vi "InjA-RT.vi"() -> ()   [LabVIEW 2016]
uses:
  Common-Control/Aperture states.ctl
  Common-Control/GP307 cluster.ctl
  Common-Control/Glassman Control.ctl
  <vilib>/FPGAPlugInAG/cRIO-9074/niLvFpga_Open_cRIO-9074.vi
  <vilib>/Utility/error.llb/Error Cluster From Error Code.vi
  <vilib>/rvi/errors/niLvFpgaAdjustHostInterfaceError.vi
  <vilib>/rvi/interface/nirviOpenFPGA/nirviOpenFPGA.xnode
  FPGA Bitfiles/Controlsoftware2_FPGATarget7_InjA-FPGA_SFV0QsfDh2c.lvbitx
  InjA-FPGA.vi
  <vilib>/rvi/interface/nirviReadWriteControl/nirviReadWriteControl.xnode
  Common-Control/Aperture Readback.ctl
  <vilib>/Instr/_visa.llb/VISA Configure Serial Port (Instr).vi
  NiFpgaLv.dll
panel:
  in  "Tab Control":T1(tab)
  out "Y Steerer Monitor.V-monitor":fxp<+/-,16,5>
  out "Y Steerer Monitor.I-monitor":fxp<+/-,16,5>
  out "X Steerer Monitor.V-monitor":fxp<+/-,16,5>
  out "X Steerer Monitor.I-monitor":fxp<+/-,16,5>
  out "Einzel 1 Monitor.I-monitor":fxp<+/-,16,5>
  out "Einzel 1 Monitor.V-monitor":fxp<+/-,16,5>
  out "Einzel 2 Monitor.V-monitor":fxp<+/-,16,5>
  out "Einzel 2 Monitor.I-monitor":fxp<+/-,16,5>
  out "Y Steerer set":T2
  out "Einzel 2 set":T2
  out "X Steerer set":T2
  out "Einzel 1 set":T2
  out "InjA Vac Cluster":T3
  out "InjA Convectron":dbl
  out "InjA Ion Gauge":dbl
  out "Ion Gauge 1":u8[](array[numeric])
  out "Convectron 1":u8[](array[numeric])
  out "Ion Gauge 2":u8[](array[numeric])
  out "Convectron 2":u8[](array[numeric])
  out "Turbo Error Status":bool
  out "Turbo Rotation Status":bool
  out "Turbo Rotation Speed":dbl
  out "Vacuum Gauge interlock":bool
  out "Pre-Acc Image  Aperture Position 2":cluster{"IN sensor":bool, "OUT sensor":bool}
  out "Pre-Acc Image  Aperture Position":T4
  out "BPM 2":bool
  out "BPM 2 x10":bool
  out "Vac cluster loop error":errorcluster
  out "HV control loop error":errorcluster
  out "Turbo readback loop error":errorcluster
  out "HV readback loop error":errorcluster
  out "Acuator-Sensor loop error":errorcluster
  out "error out":errorcluster
  out "source cage Ion gauge Cluster 2":T5={"beam line pressure  Gauge "="9.90E+09\r\n", "Turbo convectorn Gauge "="0.00E+00\r\n", "Steerer Convectro Gauge "="2.40E-08\r\n", "Ion gauge2"="7.60E-01\r\n"}
  out "element":string="0.00E+00\r\n"
  out "read buffer":string="0.00E+00\r\n"
  out "Error Reporter":errorcluster
  in  "source cage Ion gauge Cluster 4":T5
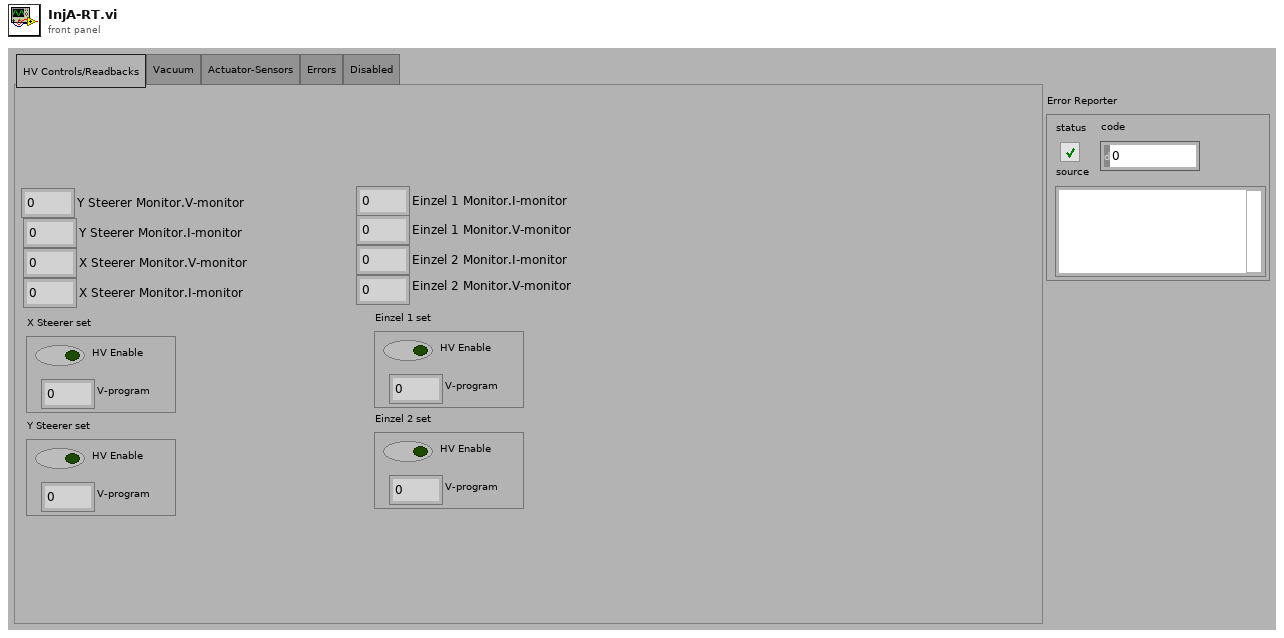
[diagram p1: front panel]
types:
  T1 = enum32{"HV Controls/Readbacks", "Vacuum", "Actuator-Sensors", "Errors", "Disabled"}
  T2 = typedef "Glassman Control.ctl" = cluster{"V-program":fxp<+/-,16,5>, "HV Enable":bool}
  T3 = typedef "GP307 cluster.ctl" = cluster{"Ion gauge 1":string, "Convectron  Gauge 1 ":string, "Ion Gauge 2":string, "Convectrom Gauge 2":string}
  T4 = typedef "Aperture states.ctl" = enum16{"Aperture status unclear", "Aperture in", "Aperture out"}
  T5 = cluster{"beam line pressure  Gauge ":string, "Turbo convectorn Gauge ":string, "Steerer Convectro Gauge ":string, "Ion gauge2":string}
  T6 = typedef "Aperture Readback.ctl" = cluster{"IN sensor":bool, "OUT sensor":bool}
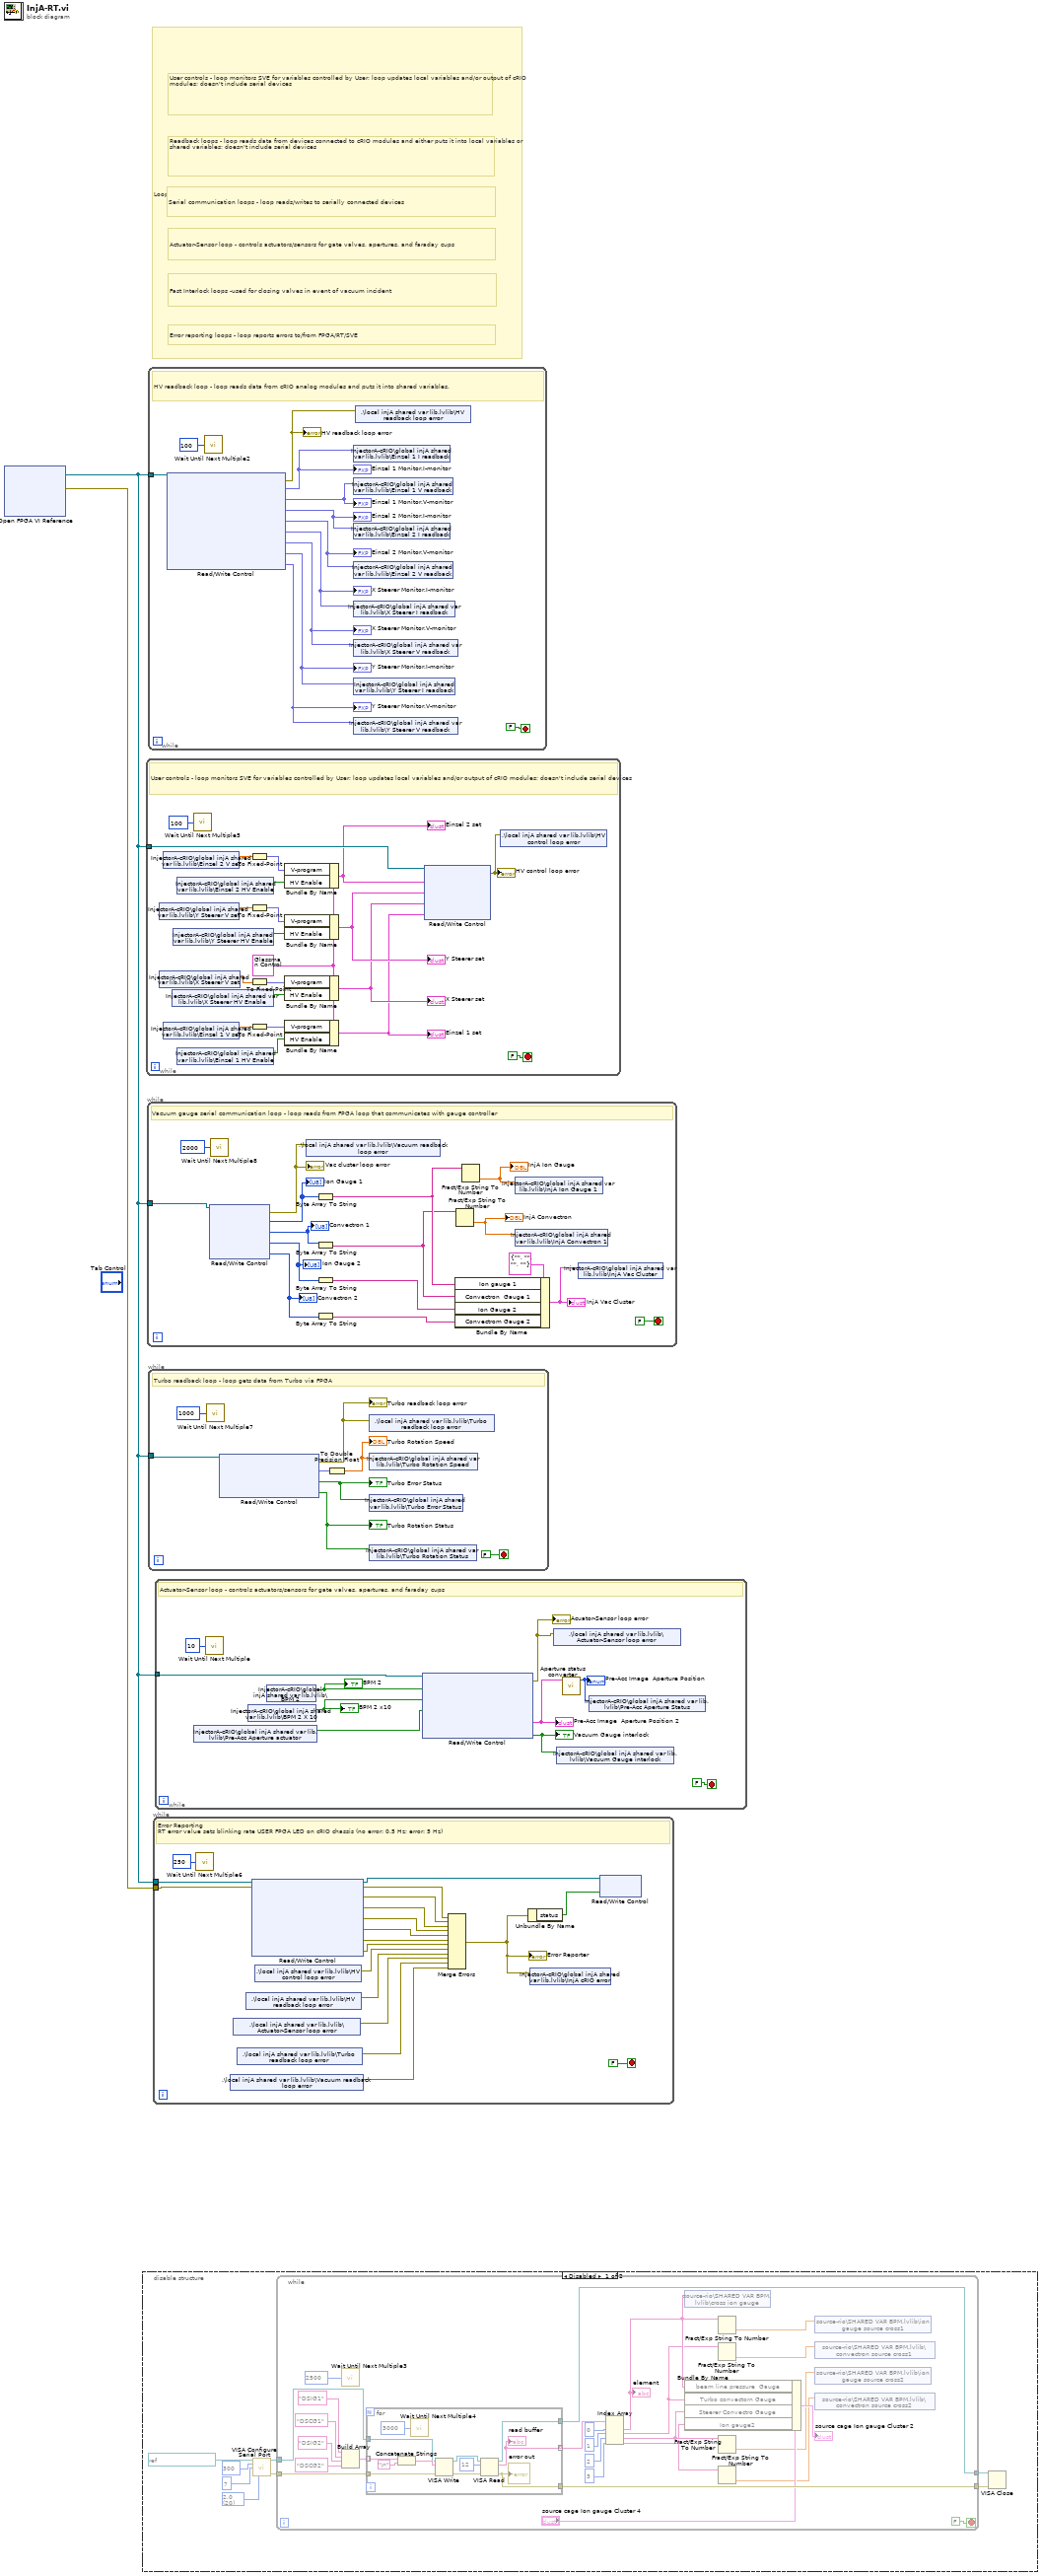
[diagram p0: block diagram]
diagram:
  # "Serial communication loops - loop reads/writes to serially connected devices"
  # "Actuator-Sensor loop - controls actuators/sensors for gate valves, apertures, and faraday cups"
  # "Fast Interlock loops -used for closing valves in event of vacuum incident"
  # "Error reporting loops - loop reports errors to/from FPGA/RT/SVE"
  # "Readback loops - loop reads data from devices connected to cRIO modules and either puts it into local variables or shared variables; doesn't include serial devices"
  # "User controls - loop monitors SVE for variables controlled by User; loop updates local variables and/or output of cRIO modules; doesn't include serial devices"
  # "Loop legend - loops are color coded by responsibility"
  n1 = xnode "Open FPGA VI Reference"() -> ("FPGA VI Reference Out"=w1:refnum<k20>, "error out"=w2:errorcluster)  [unwired: 2 in]
  n2 = disable-structure shown="Disabled" {
    frame Disabled {
      w7 = u16 20 items=["1.0"=10, "1.5"=15, "2.0"=20] ("stop bits (10: 1 bit)")
      n3 = call-poly "VISA Configure Serial Port"("VISA resource name"=refnum<visa-resource-name> "ASRL1::INSTR", "baud rate (9600)"=u32 300, "data bits (8)"=u16 7, "stop bits (10: 1 bit)"=w7) -> ("VISA resource name out"=w6:refnum<visa-resource-name>, "error out"=w5:errorcluster)  [unwired: 10 in]
      n4 = while {
        tunnel: w6 -> [w33]
        tunnel: w5 -> [w32]
        tunnel: [w31] -> w4
        tunnel: [w30] -> w3
        stop <- FALSE stop-if-true
        n5 = call "Wait Until Next Multiple3"("Count(mSec)"=u32 2500) -> ()  [unwired: 1 out]
        n6 = Build Array("DSIG1" ("write buffer"), "DSCG1" ("write buffer"), "DSIG2" ("write buffer"), "DSCG2" ("write buffer")) -> (w34:string[])
        n7 = for {
          tunnel: w34 -> [w44] mode=indexing
          tunnel: w33 -> [w42]
          tunnel: w32 -> [w41]
          tunnel: [w40] -> w29 mode=indexing
          tunnel: [w39] -> w31
          tunnel: [w38] -> w30
          n8 = Concatenate Strings(w44, "\n") -> (w43:string)
          n9 = call "Wait Until Next Multiple4"("Count(mSec)"=u32 3000) -> ()  [unwired: 1 out]
          n10 = VISA Write(VISA resource name=w42, write buffer=w43, error in (no error)=w41) -> (VISA resource name out=w47:refnum<visa-resource-name>, error out=w46:errorcluster)  [unwired: 1 out]
          n11 = VISA Read(VISA resource name=w47, byte count=u32 12, error in (no error)=w46) -> (VISA resource name out=w38:refnum<visa-resource-name>, read buffer=w40:string, error out=w39:errorcluster)  [unwired: 1 out]
          "error out" <- w39
          "read buffer" <- w40
        }
        n12 = Index Array(array=w29, index #1=0 ("index"), index #2=1 ("index"), index #3=2 ("index"), index #4=3 ("index")) -> (element #1=w18:string, element #2=w17:string, element #3=w16:string, element #4=w15:string)
        "element" <- w18
        n13 = shared-variable "source-rio\\SHARED VAR BPM.lvlib\\cross ion gauge"(w18) -> ()  [unwired: 1 in, 1 out]
        n14 = Bundle By Name(cluster="source cage Ion gauge Cluster 4", "beam line pressure  Gauge"=w18, "Turbo convectorn Gauge"=w17, "Steerer Convectro Gauge"=w16, "Ion gauge2"=w15) -> (→"source cage Ion gauge Cluster 2":T5)
        n15 = Fract/Exp String To Number(string=w18) -> (number=w14:dbl)  [unwired: 3 in, 1 out]
        n16 = Fract/Exp String To Number(string=w17) -> (number=w12:dbl)  [unwired: 3 in, 1 out]
        n17 = Fract/Exp String To Number(string=w16) -> (number=w11:dbl)  [unwired: 3 in, 1 out]
        n18 = Fract/Exp String To Number(string=w15) -> (number=w13:dbl)  [unwired: 3 in, 1 out]
        n19 = shared-variable "source-rio\\SHARED VAR BPM.lvlib\\ion gauge source cross1"(w14) -> ()  [unwired: 1 in, 1 out]
        n20 = shared-variable "source-rio\\SHARED VAR BPM.lvlib\\convectron source cross1"(w12) -> ()  [unwired: 1 in, 1 out]
        n21 = shared-variable "source-rio\\SHARED VAR BPM.lvlib\\ion gauge source cross2"(w11) -> ()  [unwired: 1 in, 1 out]
        n22 = shared-variable "source-rio\\SHARED VAR BPM.lvlib\\convectron source cross2"(w13) -> ()  [unwired: 1 in, 1 out]
      }
      n23 = VISA Close(VISA resource name=w3, error in (no error)=w4) -> ()  [unwired: 1 out]
    }
    frame Enabled {
    }
  }
  n24 = while {
    tunnel: w1 -> [w67]
    stop <- FALSE stop-if-true
    w66 = T2 {"V-program"=0.0, "HV Enable"=FALSE} ("Glassman Control")
    # "User controls - loop monitors SVE for variables controlled by User; loop updates local variables and/or output of cRIO modules; doesn't include serial devices"
    n25 = shared-variable "InjectorA-cRIO\\global injA shared var lib.lvlib\\Y Steerer V set"() -> (w63:dbl)  [unwired: 1 in, 1 out]
    n26 = shared-variable "InjectorA-cRIO\\global injA shared var lib.lvlib\\X Steerer V set"() -> (w61:dbl)  [unwired: 1 in, 1 out]
    n27 = shared-variable "InjectorA-cRIO\\global injA shared var lib.lvlib\\Einzel 2 V set"() -> (w65:dbl)  [unwired: 1 in, 1 out]
    n28 = shared-variable "InjectorA-cRIO\\global injA shared var lib.lvlib\\Einzel 1 V set"() -> (w59:dbl)  [unwired: 1 in, 1 out]
    n29 = shared-variable "InjectorA-cRIO\\global injA shared var lib.lvlib\\X Steerer HV Enable"() -> (w56:bool)  [unwired: 1 in, 1 out]
    n30 = shared-variable "InjectorA-cRIO\\global injA shared var lib.lvlib\\Y Steerer HV Enable"() -> (w55:bool)  [unwired: 1 in, 1 out]
    n31 = shared-variable "InjectorA-cRIO\\global injA shared var lib.lvlib\\Einzel 2 HV Enable"() -> (w54:bool)  [unwired: 1 in, 1 out]
    n32 = shared-variable "InjectorA-cRIO\\global injA shared var lib.lvlib\\Einzel 1 HV Enable"() -> (w57:bool)  [unwired: 1 in, 1 out]
    n33 = call "Wait Until Next Multiple5"("Count(mSec)"=u32 100) -> ()  [unwired: 1 out]
    n34 = To Fixed-Point(number=w65) -> (fixed-point=w64:fxp<+/-,16,5>)  [unwired: 1 in]
    n35 = To Fixed-Point(number=w63) -> (fixed-point=w62:fxp<+/-,16,5>)  [unwired: 1 in]
    n36 = To Fixed-Point(number=w61) -> (fixed-point=w60:fxp<+/-,16,5>)  [unwired: 1 in]
    n37 = To Fixed-Point(number=w59) -> (fixed-point=w58:fxp<+/-,16,5>)  [unwired: 1 in]
    n38 = Bundle By Name(cluster=w66, "V-program"=w64, "HV Enable"=w54) -> (w53:T2)
    "Einzel 2 set" <- w53
    n39 = Bundle By Name(cluster=w66, "V-program"=w62, "HV Enable"=w55) -> (w52:T2)
    "Y Steerer set" <- w52
    n40 = Bundle By Name(cluster=w66, "V-program"=w60, "HV Enable"=w56) -> (w51:T2)
    "X Steerer set" <- w51
    n41 = Bundle By Name(cluster=w66, "V-program"=w58, "HV Enable"=w57) -> (w50:T2)
    "Einzel 1 set" <- w50
    n42 = xnode "Read/Write Control"("FPGA VI Reference In"=w67, "Einzel 2 V set"=w53, "Y Steerer V set"=w52, "X Steerer V set"=w51, "Einzel 1 V set"=w50) -> ("error out"=w49:errorcluster)  [unwired: 1 in, 1 out]
    "HV control loop error" <- w49
    n43 = shared-variable ".\\local injA shared var lib.lvlib\\HV control loop error"(w49) -> ()  [unwired: 1 in, 1 out]
  }
  n44 = while {
    tunnel: w1 -> [w85]
    stop <- FALSE stop-if-true
    # "Vacuum gauge serial communication loop - loop reads from FPGA loop that communicates with gauge controller"
    n45 = xnode "Read/Write Control"("FPGA VI Reference In"=w85) -> ("error out"=w80:errorcluster, "Ion gauge 1"=w84:u8[], "Convectron 1"=w83:u8[], "Ion gauge 2"=w82:u8[], "Convectron 2"=w81:u8[])  [unwired: 1 in, 1 out]
    "Ion Gauge 1" <- w84
    "Convectron 1" <- w83
    "Ion Gauge 2" <- w82
    "Convectron 2" <- w81
    "Vac cluster loop error" <- w80
    n46 = call "Wait Until Next Multiple8"("Count(mSec)"=u32 2000) -> ()  [unwired: 1 out]
    n47 = shared-variable ".\\local injA shared var lib.lvlib\\Vacuum readback loop error"(w80) -> ()  [unwired: 1 in, 1 out]
    n48 = Byte Array To String(unsigned byte array=w84) -> (string=w74:string)
    n49 = Byte Array To String(unsigned byte array=w83) -> (string=w72:string)
    n50 = Byte Array To String(unsigned byte array=w82) -> (string=w71:string)
    n51 = Byte Array To String(unsigned byte array=w81) -> (string=w73:string)
    n52 = Bundle By Name(cluster=T3 {"Ion gauge 1"="", "Convectron  Gauge 1 "="", "Ion Gauge 2"="", "Convectrom Gauge 2"=""} ("Ion gauge cluster control"), "Ion gauge 1"=w74, "Convectron  Gauge 1"=w72, "Ion Gauge 2"=w71, "Convectrom Gauge 2"=w73) -> (w77:T3)
    "InjA Vac Cluster" <- w77
    n53 = Fract/Exp String To Number(string=w72) -> (number=w76:dbl)  [unwired: 3 in, 1 out]
    "InjA Convectron" <- w76
    n54 = Fract/Exp String To Number(string=w74) -> (number=w75:dbl)  [unwired: 3 in, 1 out]
    "InjA Ion Gauge" <- w75
    n55 = shared-variable "InjectorA-cRIO\\global injA shared var lib.lvlib\\InjA Ion Gauge 1"(w75) -> ()  [unwired: 1 in, 1 out]
    n56 = shared-variable "InjectorA-cRIO\\global injA shared var lib.lvlib\\InjA Convectron 1"(w76) -> ()  [unwired: 1 in, 1 out]
    n57 = shared-variable "InjectorA-cRIO\\global injA shared var lib.lvlib\\InjA Vac Cluster"(w77) -> ()  [unwired: 1 in, 1 out]
  }
  n58 = while {
    tunnel: w1 -> [w97]
    stop <- FALSE stop-if-true
    # "HV readback loop - loop reads data from cRIO analog modules and puts it into shared variables."
    n59 = xnode "Read/Write Control"("FPGA VI Reference In"=w97) -> ("error out"=w86:errorcluster, "Einzel 1 Monitor.I-monitor"=w93:fxp<+/-,16,5>, "Einzel 1 Monitor.V-monitor"=w94:fxp<+/-,16,5>, "Einzel 2 Monitor.I-monitor"=w92:fxp<+/-,16,5>, "Einzel 2 Monitor.V-monitor"=w91:fxp<+/-,16,5>, "X Steerer Monitor.I-monitor"=w88:fxp<+/-,16,5>, "X Steerer Monitor.V-monitor"=w90:fxp<+/-,16,5>, "Y Steerer Monitor.I-monitor"=w87:fxp<+/-,16,5>, "Y Steerer Monitor.V-monitor"=w89:fxp<+/-,16,5>)  [unwired: 1 in, 1 out]
    "HV readback loop error" <- w86
    "Einzel 1 Monitor.I-monitor" <- w93
    "Einzel 1 Monitor.V-monitor" <- w94
    "Y Steerer Monitor.V-monitor" <- w89
    "Y Steerer Monitor.I-monitor" <- w87
    "X Steerer Monitor.V-monitor" <- w90
    "X Steerer Monitor.I-monitor" <- w88
    "Einzel 2 Monitor.V-monitor" <- w91
    "Einzel 2 Monitor.I-monitor" <- w92
    n60 = call "Wait Until Next Multiple2"("Count(mSec)"=u32 100) -> ()  [unwired: 1 out]
    n61 = shared-variable "InjectorA-cRIO\\global injA shared var lib.lvlib\\Einzel 1 I readback"(w93) -> ()  [unwired: 1 in, 1 out]
    n62 = shared-variable "InjectorA-cRIO\\global injA shared var lib.lvlib\\Einzel 1 V readback"(w94) -> ()  [unwired: 1 in, 1 out]
    n63 = shared-variable "InjectorA-cRIO\\global injA shared var lib.lvlib\\Einzel 2 I readback"(w92) -> ()  [unwired: 1 in, 1 out]
    n64 = shared-variable "InjectorA-cRIO\\global injA shared var lib.lvlib\\Einzel 2 V readback"(w91) -> ()  [unwired: 1 in, 1 out]
    n65 = shared-variable "InjectorA-cRIO\\global injA shared var lib.lvlib\\X Steerer I readback"(w88) -> ()  [unwired: 1 in, 1 out]
    n66 = shared-variable "InjectorA-cRIO\\global injA shared var lib.lvlib\\X Steerer V readback"(w90) -> ()  [unwired: 1 in, 1 out]
    n67 = shared-variable "InjectorA-cRIO\\global injA shared var lib.lvlib\\Y Steerer I readback"(w87) -> ()  [unwired: 1 in, 1 out]
    n68 = shared-variable "InjectorA-cRIO\\global injA shared var lib.lvlib\\Y Steerer V readback"(w89) -> ()  [unwired: 1 in, 1 out]
    n69 = shared-variable ".\\local injA shared var lib.lvlib\\HV readback loop error"(w86) -> ()  [unwired: 1 in, 1 out]
  }
  n70 = while {
    tunnel: w1 -> [w105]
    stop <- FALSE stop-if-true
    # "Turbo readback loop - loop gets data from Turbo via FPGA"
    n71 = call "Wait Until Next Multiple7"("Count(mSec)"=u32 1000) -> ()  [unwired: 1 out]
    n72 = xnode "Read/Write Control"("FPGA VI Reference In"=w105) -> ("error out"=w99:errorcluster, "Turbo Rotation Speed"=w103:fxp<+/-,26,5>, "Turbo Error Status"=w102:bool, "Turbo Rotation Status"=w101:bool)  [unwired: 1 in, 1 out]
    "Turbo Error Status" <- w102
    "Turbo Rotation Status" <- w101
    "Turbo readback loop error" <- w99
    n73 = To Double Precision Float(number=w103) -> (double precision float=w100:dbl)
    "Turbo Rotation Speed" <- w100
    n74 = shared-variable ".\\local injA shared var lib.lvlib\\Turbo readback loop error"(w99) -> ()  [unwired: 1 in, 1 out]
    n75 = shared-variable "InjectorA-cRIO\\global injA shared var lib.lvlib\\Turbo Rotation Speed"(w100) -> ()  [unwired: 1 in, 1 out]
    n76 = shared-variable "InjectorA-cRIO\\global injA shared var lib.lvlib\\Turbo Error Status"(w102) -> ()  [unwired: 1 in, 1 out]
    n77 = shared-variable "InjectorA-cRIO\\global injA shared var lib.lvlib\\Turbo Rotation Status"(w101) -> ()  [unwired: 1 in, 1 out]
  }
  n78 = while {
    tunnel: w1 -> [w122]
    tunnel: w2 -> [w121]
    stop <- FALSE stop-if-true
    # "Error Reporting\nRT error value sets blinking rate USER FPGA LED on cRIO chassis (no error: 0.5 Hz; error: 5 Hz)"
    n79 = call "Wait Until Next Multiple6"("Count(mSec)"=u32 250 ("millisecond multiple")) -> ()  [unwired: 1 out]
    n80 = shared-variable ".\\local injA shared var lib.lvlib\\Vacuum readback loop error"() -> (w106:errorcluster)  [unwired: 1 in, 1 out]
    n81 = shared-variable ".\\local injA shared var lib.lvlib\\Actuator-Sensor loop error"() -> (w108:errorcluster)  [unwired: 1 in, 1 out]
    n82 = shared-variable ".\\local injA shared var lib.lvlib\\Turbo readback loop error"() -> (w107:errorcluster)  [unwired: 1 in, 1 out]
    n83 = shared-variable ".\\local injA shared var lib.lvlib\\HV readback loop error"() -> (w109:errorcluster)  [unwired: 1 in, 1 out]
    n84 = xnode "Read/Write Control"("FPGA VI Reference In"=w122, "error in"=w121) -> ("FPGA VI Reference Out"=w112:refnum<k20>, "error out"=w120:errorcluster, "Actuator Sensor loop error"=w119:errorcluster, "Vac Interlock loop error"=w118:errorcluster, "Vac readback loop error"=w117:errorcluster, "HV readback loop error"=w116:errorcluster, "HV control loop error"=w115:errorcluster, "Turbo monitor loop error"=w114:errorcluster)
    n85 = shared-variable ".\\local injA shared var lib.lvlib\\HV control loop error"() -> (w110:errorcluster)  [unwired: 1 in, 1 out]
    n86 = Merge Errors(w120, w119, w118, w117, w116, w115, w114, w110, w109, w108, w107, w106) -> (w113:errorcluster)
    "Error Reporter" <- w113
    n87 = Unbundle By Name(w113) -> ("status"=w111:bool)
    n88 = shared-variable "InjectorA-cRIO\\global injA shared var lib.lvlib\\InjA cRIO error"(w113) -> ()  [unwired: 1 in, 1 out]
    n89 = xnode "Read/Write Control"("FPGA VI Reference In"=w112, "RT error"=w111) -> ()  [unwired: 1 in, 2 out]
  }
  n90 = while {
    tunnel: w1 -> [w134]
    stop <- FALSE stop-if-true
    # "Actuator-Sensor loop - controls actuators/sensors for gate valves, apertures, and faraday cups"
    n91 = shared-variable "InjectorA-cRIO\\global injA shared var lib.lvlib\\Pre-Acc Aperture actuator"() -> (w127:bool)  [unwired: 1 in, 1 out]
    n92 = call "Wait Until Next Multiple"("Count(mSec)"=u32 10) -> ()  [unwired: 1 out]
    n93 = shared-variable "InjectorA-cRIO\\global injA shared var lib.lvlib\\BPM 2 X 10"() -> (w131:bool)  [unwired: 1 in, 1 out]
    "BPM 2 x10" <- w131
    n94 = shared-variable "InjectorA-cRIO\\global injA shared var lib.lvlib\\BPM 2"() -> (w130:bool)  [unwired: 1 in, 1 out]
    "BPM 2" <- w130
    n95 = xnode "Read/Write Control"("FPGA VI Reference In"=w134, "BPM 2"=w130, "BPM 2x10"=w131, "Pre-Acc Aperture Actuator"=w127) -> ("error out"=w125:errorcluster, "Pre-Acc Aperture Position"=w128:T6, "Vacuum Gauge interlock"=w126:bool)  [unwired: 1 in, 1 out]
    "Pre-Acc Image  Aperture Position 2" <- w128
    "Vacuum Gauge interlock" <- w126
    "Acuator-Sensor loop error" <- w125
    n96 = shared-variable ".\\local injA shared var lib.lvlib\\Actuator-Sensor loop error"(w125) -> ()  [unwired: 1 in, 1 out]
    n97 = shared-variable "InjectorA-cRIO\\global injA shared var lib.lvlib\\Vacuum Gauge interlock"(w126) -> ()  [unwired: 1 in, 1 out]
    n98 = call "Aperture status converter.vi"("Aperture Position"=w128) -> ("Aperture Status"=w129:T4)  [unwired: 10 in]
    "Pre-Acc Image  Aperture Position" <- w129
    n99 = shared-variable "InjectorA-cRIO\\global injA shared var lib.lvlib\\Pre-Acc Aperture Status"(w129) -> ()  [unwired: 1 in, 1 out]
  }
